vi "Asylum_XOPVersion.vi"(8 "error in (no error)":errorcluster, 11 "Application":refnum<k7>) -> (0 "error out":errorcluster, 2 "results":string, 3 "Application":refnum<k7>)   [LabVIEW 2019]
doc: "Returns a string containing the version number of the MFP3D Xop."
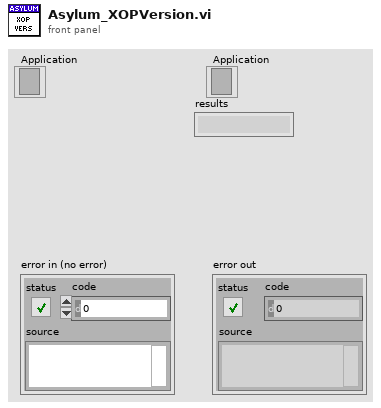
[diagram p1: front panel]
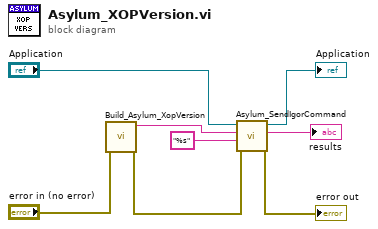
[diagram p0: block diagram]
diagram:
  n1 = call "Build_Asylum_XopVersion.vi"("error in (no error)"="error in (no error)") -> ("error out"=w8:errorcluster, "Command"=w6:string)  [unwired: 9 in]
  n2 = call "Asylum_SendIgorCommand.vi"("error in (no error)"=w8, "Format"="%s", "command"=w6, "Application In"="Application") -> ("error out"=→"error out":errorcluster, "results"=→"results":string, "Application Out"=→"Application":refnum<k7>)  [unwired: 4 in, 1 out]
